vi "vectornav RT test PC.vi"() -> ()   [LabVIEW 2009]
uses:
  <vilib>/Instr/_visa.llb/VISA Configure Serial Port (Instr).vi
  vectornav data.vi
panel:
  in  "stop":bool
  in  "VISA resource name":refnum<visa-resource-name>
  out "z-magnetic":dbl
  out "y-magnetic":dbl
  out "x-magnetic":dbl
  out "y-acceleration 2":dbl
  out "y-acceleration":dbl
  out "x-acceleration":dbl
  out "q[3]":dbl
  out "q[2]":dbl
  out "q[1]":dbl
  out "q[0]":dbl
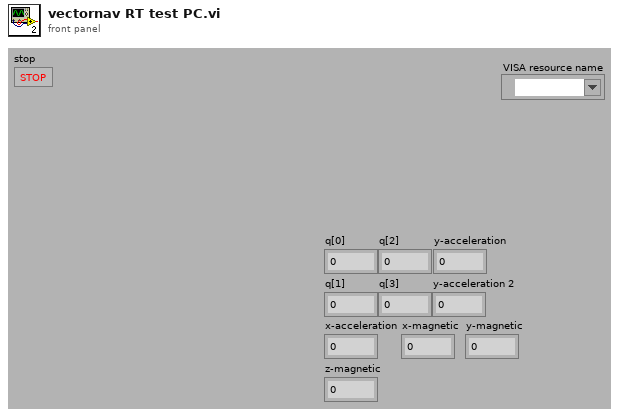
[diagram p1: front panel]
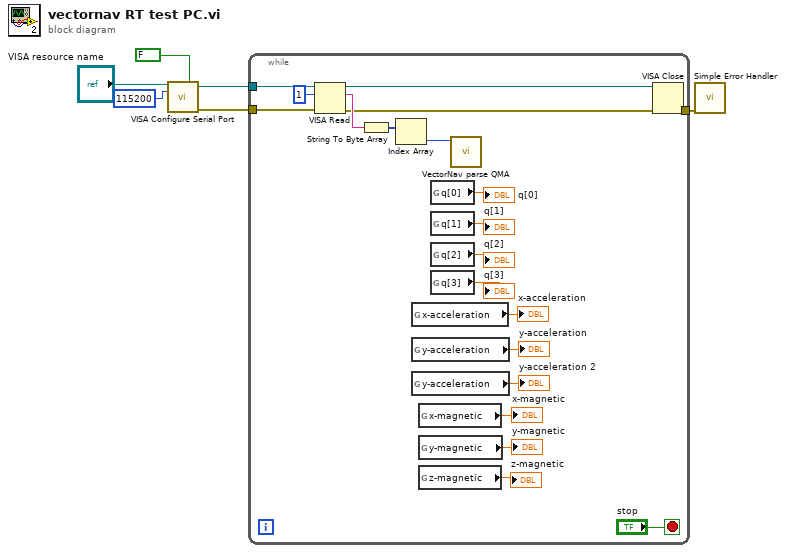
[diagram p0: block diagram]
diagram:
  n1 = call-poly "VISA Configure Serial Port"("VISA resource name"="VISA resource name", "Enable Termination\nChar (T)"=FALSE ("Enable Termination\nChar (T)"), "baud rate (9600)"=u32 115200) -> ("VISA resource name out"=w2:refnum<visa-resource-name>, "error out"=w3:errorcluster)  [unwired: 11 in]
  n2 = while {
    tunnel: w3 -> [w13]
    tunnel: w2 -> [w12]
    tunnel: [w11] -> w1
    stop <- "stop" stop-if-true
    n3 = VISA Read(VISA resource name=w12, byte count=u32 1, error in (no error)=w13) -> (VISA resource name out=w9:refnum<visa-resource-name>, read buffer=w16:string, error out=w10:errorcluster)  [unwired: 1 out]
    n4 = String To Byte Array(string=w16) -> (unsigned byte array=w15:u8[])
    n5 = Index Array(array=w15) -> (element=w14:u8)  [unwired: 1 in]
    n6 = global read "vectornav data.vi" "x-acceleration"() -> (→"x-acceleration":dbl)
    n7 = global read "vectornav data.vi" "y-acceleration"() -> (→"y-acceleration":dbl)
    n8 = global read "vectornav data.vi" "y-acceleration"() -> (→"y-acceleration 2":dbl)
    n9 = global read "vectornav data.vi" "x-magnetic"() -> (→"x-magnetic":dbl)
    n10 = global read "vectornav data.vi" "y-magnetic"() -> (→"y-magnetic":dbl)
    n11 = global read "vectornav data.vi" "z-magnetic"() -> (→"z-magnetic":dbl)
    n12 = global read "vectornav data.vi" "q[0]"() -> (→"q[0]":dbl)
    n13 = global read "vectornav data.vi" "q[1]"() -> (→"q[1]":dbl)
    n14 = global read "vectornav data.vi" "q[2]"() -> (→"q[2]":dbl)
    n15 = global read "vectornav data.vi" "q[3]"() -> (→"q[3]":dbl)
    n16 = call "VectorNav parse QMA.vi"("input data"=w14) -> ()  [unwired: 11 in]
    n17 = VISA Close(VISA resource name=w9, error in (no error)=w10) -> (error out=w11:errorcluster)
  }
  n18 = call <vilib>:"Simple Error Handler.vi"("error in (no error)"=w1) -> ()  [unwired: 4 in, 5 out]
